vi "Ensure File Exists.vi"(8 "error in":errorcluster, 11 "Approved":path) -> (0 "error out":errorcluster, 3 "File Path":path)   [LabVIEW 2020, in "Approval Tests.lvlib"]
uses:
  Approval Tests.lvlib
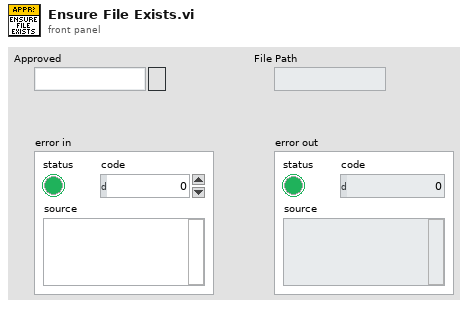
[diagram p1: front panel]
types:
  T1 = enum32{"invalid VI type", "Standard VI", "Control VI", "Global VI", "Polymorphic VI", "Configuration VI", "SubSystem", "Facade VI", "Method VI", "Statechart Diagram VI"}
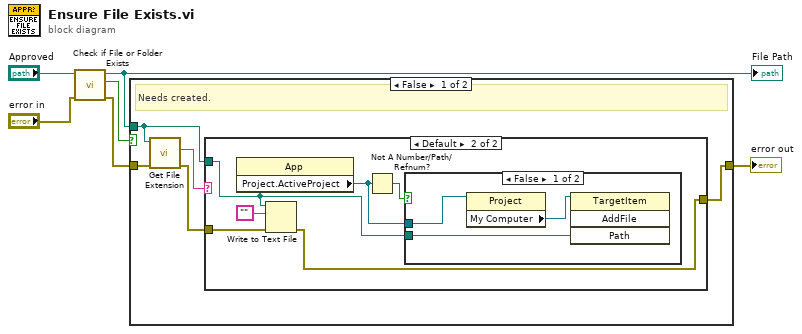
[diagram p0: block diagram]
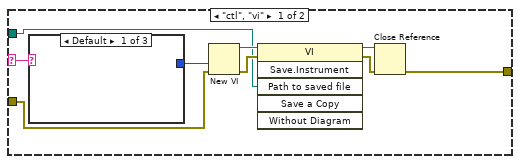
[diagram p2: hidden frame]
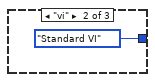
[diagram p3: hidden frame]
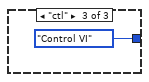
[diagram p4: hidden frame]
diagram:
  n1 = call <vilib>:"Check if File or Folder Exists.vi"("error in (no error)"="error in", "path"="Approved") -> ("error out"=w5:errorcluster, "file or folder exists?"=w2:bool, "dup path"=w1:path)  [unwired: 7 in]
  "File Path" <- w1
  n2 = case shown="False" w2 {
    tunnel: w5 -> [w10 w32]
    tunnel: [w11 w32] -> w4
    tunnel: w1 -> [w7 _]
    frame False {
      # "Needs created."
      n3 = call <vilib>:"Get File Extension.vi"("error in (no error)"=w10, "file"=w7) -> ("error out"=w9:errorcluster, "lowercase file extension"=w8:string)  [unwired: 5 in, 3 out]
      n4 = case shown="Default" w8 {
        selector: w8 -> [w12 _]
        tunnel: [w17 w28] -> w11
        tunnel: w7 -> [w14 w23]
        tunnel: w9 -> [w20 w27]
        frame "ctl", "vi" {
          n5 = case shown="Default" w12 {
            tunnel: [_ T1."Standard VI" ("vi type (standard vi)") T1."Control VI" ("vi type (standard vi)")] -> w13
            frame Default {
            }
            frame "vi" {
            }
            frame "ctl" {
            }
          }
          n6 = New VI(8:w20, 9:w13) -> (0:w19:errorcluster, 3:w16:refnum<vi>)  [unwired: 5 in]
          n7 = invoke class="VI" method="Save.Instrument"(reference=w16, error in=w19, "Path to saved file"=w14) -> (reference out=w15:refnum<vi>, error out=w18:errorcluster)  [unwired: 3 in, 4 out]
          n8 = Close Reference(reference=w15, error in (no error)=w18) -> (error out=w17:errorcluster)
        }
        frame Default {
          n9 = property class="App"() -> ("Project.ActiveProject"=w24:refnum<vi>)  [unwired: 2 in, 2 out]
          n10 = Write to Text File(file (use dialog)=w23, text="", error in=w27) -> (error out=w28:errorcluster)  [unwired: 1 in, 2 out]
          n11 = Not A Number/Path/Refnum?(number/path/refnum=w24) -> (NaN/Path/Refnum?=w25:bool)
          n12 = case shown="False" w25 {
            tunnel: w24 -> [w31 _]
            tunnel: w23 -> [w30 _]
            frame False {
              n13 = property class="Project"(reference=w31) -> ("My Computer"=w29:refnum<vi>)  [unwired: 1 in, 2 out]
              n14 = invoke class="TargetItem" method="AddFile"(reference=w29, "Path"=w30) -> ()  [unwired: 2 in, 4 out]
            }
            frame True {
            }
          }
        }
      }
    }
    frame True {
      # "Does exist"
    }
  }
  "error out" <- w4
